vi "F to C.vi"(11 "fahrenheit":dbl) -> (3 "celsius":dbl)   [LabVIEW 2019, in "Temperature Controller.lvclass"]
uses:
  Temperature Controller.lvclass
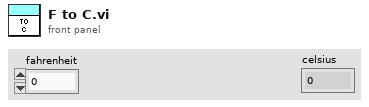
[diagram p1: front panel]
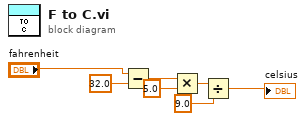
[diagram p0: block diagram]
diagram:
  n1 = Subtract(x="fahrenheit", y=32.0) -> (x-y=w5:dbl)
  n2 = Multiply(x=w5, y=5.0) -> (x*y=w3:dbl)
  n3 = Divide(x=w3, y=9.0) -> (x/y=→"celsius":dbl)
